vi "SIM Get Real LUP Matrix.vi"(0 "LU Info":cluster{"LU":dbl[][], "Pivot":i32[]} {"LU" format="%.3f"}) -> (1 "L":T1, 2 "U":T1, 3 "P":i32[][](array[numeric]))   [LabVIEW 2018]
uses:
  RealMatrix.ctl
  <resource>/lvanlys.dll
  NI_Matrix.lvlib
panel:
  # "Get Real LUP Matrix"
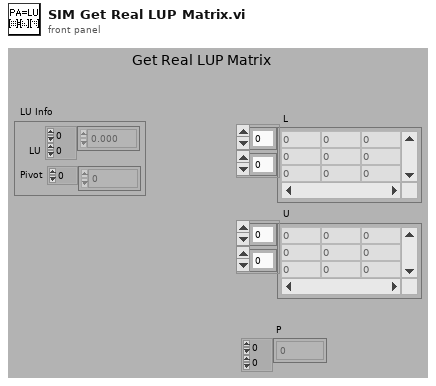
[diagram p1: front panel]
types:
  T1 = typedef "NI_Matrix.lvlib/RealMatrix.ctl" = dbl[][]
  T2 = enum32{"Identity", "Diagonal", "Toepliz", "Vandermonde", "Companion"}
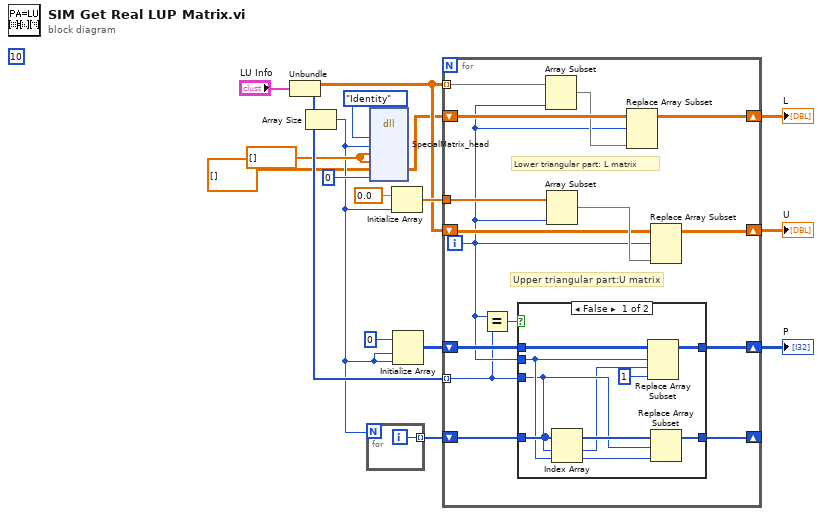
[diagram p0: block diagram]
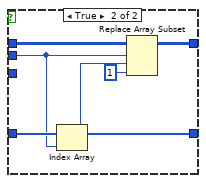
[diagram p2: hidden frame]
diagram:
  w6 = dbl[] [] ("Input Vector1")
  (unwired) 10
  n1 = Unbundle("LU Info") -> ("LU"=w15:dbl[][], "Pivot"=w11:i32[])
  n2 = Array Size(array=w11) -> (size(s)=w5:i32)
  n3 = for {
    N: w5 -> [_]
    tunnel: [w18] -> w12 mode=indexing
    i -> [w18]
  }
  n4 = dll-call lib="C:/Program Files (x86)/National Instruments/LabVIEW 2018/resource/lvanlys.*" fn="SpecialMatrix_head"("matrix type"=T2."Identity", "matrix size"=w5, "Input Vector1"=w6, "Input Vector2"=w6, "Special Matrix"=T1 [], "output param"=0) -> ("Special Matrix"=w2:T1)  [unwired: 9 in, 2 out]
  n5 = Initialize Array(0.0 ("element"), w5) -> (w16:dbl[])
  n6 = Initialize Array(0, w5, w5) -> (w13:i32[][])
  n7 = for {
    tunnel: w15 -> [w31] mode=indexing
    shift-right: [w32] -> w1
    shift-left: w2 -> [w33]
    tunnel: w16 -> [w29]
    shift-right: [w26] -> w9
    shift-left: w15 -> [w27]
    shift-right: [w25] -> w8
    shift-left: w13 -> [w24]
    shift-right: [w22] -> _
    shift-left: w12 -> [w23]
    tunnel: w11 -> [w19] mode=indexing
    i -> [w20]
    # "Upper triangular part:U matrix"
    # "Lower triangular part: L matrix"
    n8 = Equal?(x=w20, y=w19) -> (x = y?=w21:bool)
    n9 = case shown="False" w21 {
      tunnel: w23 -> [w42 w45]
      tunnel: [w41 w45] -> w22
      tunnel: w19 -> [w36 _]
      tunnel: w20 -> [w37 w44]
      tunnel: w24 -> [w40 w48]
      tunnel: [w39 w47] -> w25
      frame False {
        n10 = Index Array(array=w42, index #1=w36, index #2=w37) -> (element #1=w34:i32, element #2=w35:i32)
        n11 = Replace Array Subset(array=w40, new element=1 ("new element/subarray"), index (row)=w37, index (col)=w34) -> (w39:i32[][])
        n12 = Replace Array Subset(array=w42, new element=w35, index=w36) -> (w41:i32[])
      }
      frame True {
        n13 = Index Array(array=w45, index=w44) -> (element=w43:i32)
        n14 = Replace Array Subset(array=w48, new element=1, index (row)=w44, index (col)=w43) -> (w47:i32[][])
      }
    }
    n15 = Array Subset(array=w31, length=w20) -> (w30:dbl[])  [unwired: 1 in]
    n16 = Array Subset(array=w29, length=w20) -> (w28:dbl[])  [unwired: 1 in]
    n17 = Replace Array Subset(array=w33, new element=w30, index (row)=w20) -> (w32:T1)  [unwired: 1 in]
    n18 = Replace Array Subset(array=w27, new element=w28, index (row)=w20) -> (w26:dbl[][])  [unwired: 1 in]
  }
  "U" <- w9
  "L" <- w1
  "P" <- w8
